vi "FTW-Connector-Core-Ask-Unvalidated.vi"(0 "Actor Connector":T1, 5 "Raw Request":string="{\"FTW-Request-Header\":\"FTW-ActorStatus\"}", 9 "Timeout":i32=100 format="%dmsec", 11 "error in":errorcluster) -> (4 "Actor Connector out":T1, 6 "Raw Response":string, 15 "error out":errorcluster)   [LabVIEW 2015]
uses:
  core/type/FTW-Type-Actor-Connector.ctl
panel:
  # "Inputs"
  # "Outputs"
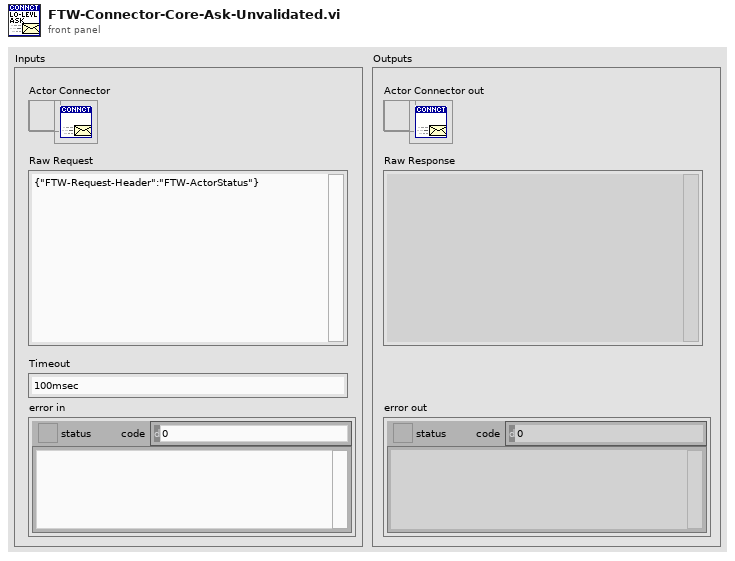
[diagram p1: front panel]
types:
  T1 = typedef "FTW-Type-Actor-Connector.ctl" = refnum<data-value>
  T2 = cluster{"FTW-CodeGen-Type":enum16{"FTW-Actor-Connector"}, "Socket":i64}
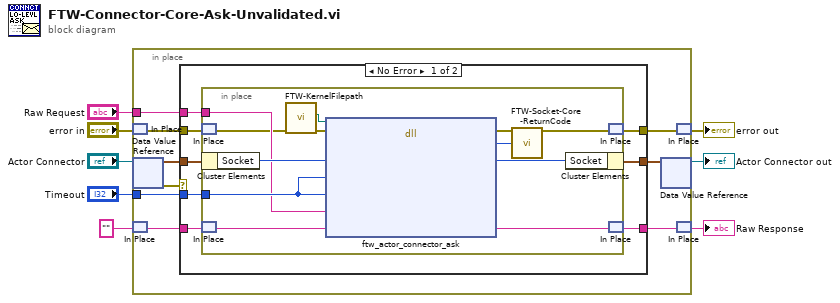
[diagram p0: block diagram]
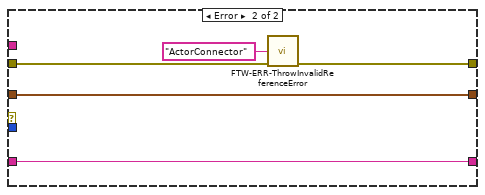
[diagram p2: hidden frame]
diagram:
  n1 = in-place {
    in-place-border: "Timeout" -> [w17]
    in-place-border: "Raw Request" -> [w16]
    n2 = in-place-match #1("error in") -> (w10:errorcluster)
    n3 = in-place-dvr #2("Actor Connector") -> (w15:T2, w13:errorcluster)
    n4 = in-place-match #3("") -> (w12:string)
    n5 = case shown="No Error" w13 {
      tunnel: w10 -> [w19 w39]
      tunnel: [w18 w38] -> w9
      tunnel: [w20 w41] -> w11
      tunnel: w17 -> [w25 _]
      tunnel: w16 -> [w24 _]
      tunnel: w15 -> [w23 w42]
      tunnel: [w22 w42] -> w14
      tunnel: w12 -> [w21 w41]
      frame No Error {
        n6 = in-place {
          in-place-border: w25 -> [w32]
          in-place-border: w24 -> [w31]
          n7 = in-place-match #4(w19) -> (w27:errorcluster)
          n8 = in-place-cluster #5(w23) -> ("Socket"=w36:i64)
          n9 = in-place-match #6(w21) -> (w29:string)
          n10 = call "FTW-KernelFilepath.vi"("error in"=w27) -> ("error out"=w34:errorcluster, "Library Filepath"=w33:path)  [unwired: 8 in, 1 out]
          n11 = dll-call lib="?" fn="ftw_actor_connector_ask"(path in=w33, error in=w34, "Socket Handle"=w36, "Send Timeout"=w32, "Recv Timeout"=w32, "Request"=w31, "Response"=w29) -> (error out=w37:errorcluster, "Return Code"=w30:i64, "Socket Handle"=w35:i64, "Response"=w28:string)  [unwired: 4 in, 1 out]
          n12 = call "FTW-Socket-Core-ReturnCode.vi"("error in"=w37, "Return Code"=w30) -> ("error out"=w26:errorcluster)  [unwired: 13 in]
          n13 = in-place-cluster #5("Socket"=w35) -> (w22:T2)
          n14 = in-place-match #4(w26) -> (w18:errorcluster)
          n15 = in-place-match #6(w28) -> (w20:string)
        }
      }
      frame Error {
        n16 = call "FTW-ERR-ThrowInvalidReferenceError.vi"("Reference Type"="ActorConnector", "error in"=w39) -> ("error out"=w38:errorcluster)  [unwired: 13 in]
      }
    }
    n17 = in-place-dvr #2(w14) -> (→"Actor Connector out":T1)  [unwired: 1 out]
    n18 = in-place-match #1(w9) -> (→"error out":errorcluster)
    n19 = in-place-match #3(w11) -> (→"Raw Response":string)
  }
